vi "credential check_19-07-16.vi"(0 "Credentials file path":path, 2 "USER NAME":string, 3 "PASSWORD":string, 5 "error in":errorcluster) -> (14 "user?":string, 15 "USER EXISTS?":bool, 16 "User Name":bool, 17 "Password":bool, 19 "error out":errorcluster)   [LabVIEW 2015]
uses:
  <vilib>/Utility/file.llb/Read Delimited Spreadsheet (string).vi
panel:
  out "all rows":string[][](array[string])
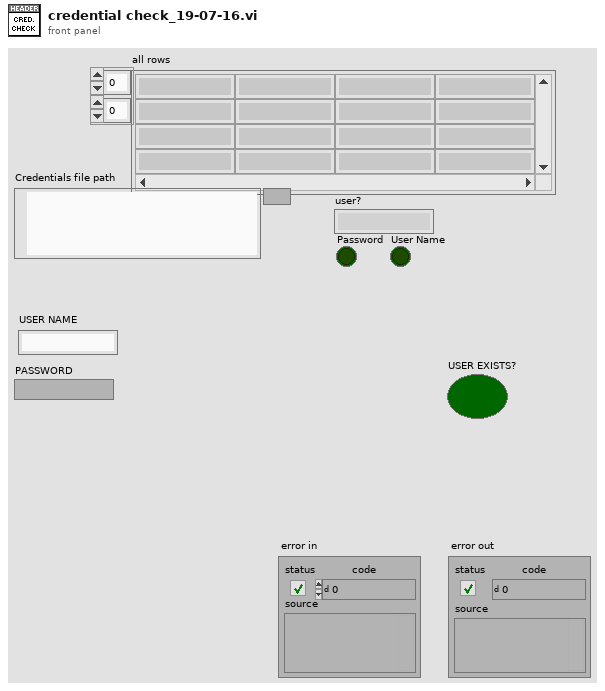
[diagram p1: front panel]
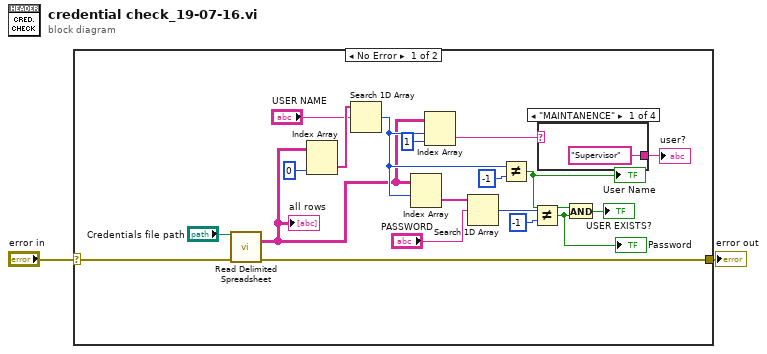
[diagram p0: block diagram]
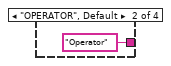
[diagram p2: hidden frame]
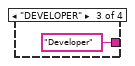
[diagram p3: hidden frame]
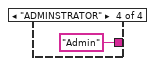
[diagram p4: hidden frame]
diagram:
  n1 = case shown="No Error" "error in" {
    selector: "error in" -> [w20 w26]
    tunnel: [w21 w26] -> w2
    frame No Error {
      n2 = call-poly <vilib>:"Read Delimited Spreadsheet.vi"("file path (dialog if empty)"="Credentials file path", "error in (no error)"=w20) -> ("all rows"=w8:string[][], "error out"=w21:errorcluster)  [unwired: 8 in, 4 out]
      "all rows" <- w8
      n3 = Index Array(array=w8, index (col)=0 ("disabled index (col)")) -> (element=w18:string[])  [unwired: 1 in]
      n4 = Search 1D Array(1D array=w18, element="USER NAME") -> (index of element=w9:i32)  [unwired: 1 in]
      n5 = Index Array(array=w8, index (row)=w9) -> (element=w12:string[])  [unwired: 1 in]
      n6 = Index Array(array=w8, index (row)=w9, index (col)=1 ("disabled index (col)")) -> (element=w6:string)
      n7 = Search 1D Array(1D array=w12, element="PASSWORD") -> (index of element=w11:i32)  [unwired: 1 in]
      n8 = Not Equal?(x=w9, y=-1) -> (x != y?=w3:bool)
      "User Name" <- w3
      n9 = Not Equal?(x=w11, y=-1) -> (x != y?=w14:bool)
      "Password" <- w14
      n10 = case shown="\"MAINTANENCE\"" w6 {
        tunnel: ["Supervisor" "Operator" "Developer" "Admin"] -> w5
        frame "MAINTANENCE" {
        }
        frame "OPERATOR", Default {
        }
        frame "DEVELOPER" {
        }
        frame "ADMINSTRATOR" {
        }
      }
      "user?" <- w5
      n11 = And(x=w3, y=w14) -> (x .and. y?=→"USER EXISTS?":bool)
    }
    frame Error {
    }
  }
  "error out" <- w2
